vi "Parse JSON Enum Values.vi"(8 "error in":errorcluster, 11 "JSON enum string":string) -> (0 "error out":errorcluster, 1 "enum items":string[](array[string]), 2 "enum items and values":cluster{"String":string, "Value":i32}[](array[cluster]), 3 "sparse enum?":bool)   [LabVIEW 2021, in "NI Measurement V2 Client Generator Runtime.lvlib"]
uses:
  NI Measurement V2 Client Generator Runtime.lvlib
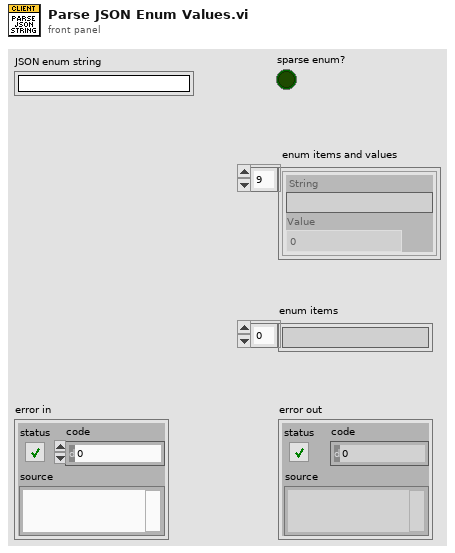
[diagram p1: front panel]
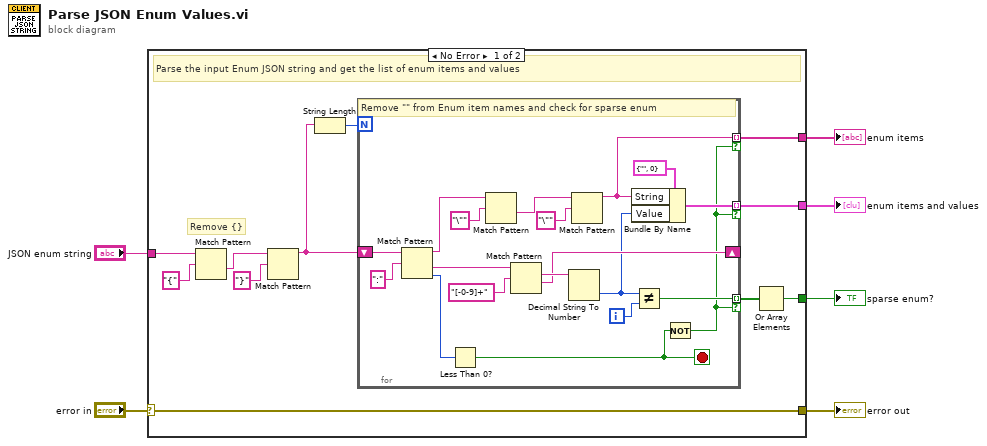
[diagram p0: block diagram]
diagram:
  n1 = case shown="No Error" "error in" {
    selector: "error in" -> [w13 w37]
    tunnel: "JSON enum string" -> [w16 _]
    tunnel: [w13 w37] -> w4
    tunnel: [w12 _] -> w3
    tunnel: [w10 _] -> w2
    tunnel: [w9 _] -> w1
    frame No Error {
      # "Remove {}"
      # "Parse the input Enum JSON string and get the list of enum items and values"
      n2 = Match Pattern(string=w16, regular expression="{") -> (after substring=w15:string)  [unwired: 1 in, 3 out]
      n3 = Match Pattern(string=w15, regular expression="}") -> (before substring=w8:string)  [unwired: 1 in, 3 out]
      n4 = String Length(string=w8) -> (length=w7:i32)
      n5 = for {
        N: w7 -> [_]
        shift-right: [w25] -> _
        shift-left: w8 -> [w36]
        tunnel: [w23] -> w11 mode=indexing if=w18
        tunnel: [w30] -> w12 mode=indexing if=w18
        tunnel: [w19] -> w9 mode=indexing if=w18
        i -> [w22]
        stop <- w24 stop-if-true
        # "Remove \"\" from Enum item names and check for sparse enum"
        n6 = Match Pattern(string=w36, regular expression=":") -> (before substring=w33:string, after substring=w21:string, offset past match=w35:i32)  [unwired: 1 in, 1 out]
        n7 = Less Than 0?(x=w35) -> (x < 0?=w24:bool)
        n8 = Match Pattern(string=w33, regular expression="\"") -> (after substring=w32:string)  [unwired: 1 in, 3 out]
        n9 = Match Pattern(string=w21, regular expression="[-0-9]+") -> (match substring=w26:string, after substring=w25:string)  [unwired: 1 in, 2 out]
        n10 = Decimal String To Number(string=w26) -> (number=w20:i32)  [unwired: 2 in, 1 out]
        n11 = Match Pattern(string=w32, regular expression="\"") -> (before substring=w19:string)  [unwired: 1 in, 3 out]
        n12 = Bundle By Name(cluster=cluster{"String":string, "Value":i32} {"String"="", "Value"=0}, "String"=w19, "Value"=w20) -> (w30:cluster{"String":string, "Value":i32})
        n13 = Not Equal?(x=w20, y=w22) -> (x != y?=w23:bool)
        n14 = Not(x=w24) -> (.not. x?=w18:bool)
      }
      n15 = Or Array Elements(Boolean array=w11) -> (logical OR=w10:bool)
    }
    frame Error {
      # "Pass"
    }
  }
  "error out" <- w4
  "sparse enum?" <- w2
  "enum items and values" <- w3
  "enum items" <- w1
